vi "dummy encoder edge detection (non-FPGA style).vi"(5 "Tick Count(Ticks)":u32, 6 "rising edge (T)":bool=TRUE, 7 "switch encoders (F)":bool, 8 "ticks":u32[](array[numeric])=[0, 0], 9 "encoder 2":bool, 10 "encoder 1":bool, 11 "history in":bool[](array[boolean])=[FALSE, FALSE, FALSE, FALSE, FALSE, FALSE, FALSE, FALSE, FALSE, FALSE, FALSE, FALSE, FALSE, FALSE, FALSE, FALSE, FALSE, FALSE, FALSE, FALSE, FALSE, FALSE, FALSE, FALSE, FALSE, FALSE, FALSE, FALSE, FALSE, FALSE, FALSE, FALSE, FALSE, FALSE, FALSE, FALSE, FALSE, FALSE, FALSE, FALSE, FALSE, FALSE, FALSE, FALSE, FALSE, FALSE, FALSE, FALSE, FALSE, FALSE, FALSE, FALSE, FALSE, FALSE, FALSE, FALSE, FALSE, FALSE, FALSE, FALSE, FALSE, FALSE, FALSE, FALSE, FALSE, FALSE, FALSE, FALSE, FALSE, FALSE, FALSE, FALSE, FALSE, FALSE, FALSE, FALSE, FALSE, FALSE, FALSE, FALSE, FALSE, FALSE, FALSE, FALSE, FALSE, FALSE, FALSE, FALSE, FALSE, FALSE, FALSE, FALSE, FALSE, FALSE, FALSE, FALSE, FALSE, FALSE, FALSE, FALSE]) -> (0 "ticks out":u32[](array[numeric]), 1 "edge detected":bool, 3 "history out":bool[](array[boolean]))   [LabVIEW 2018]
panel:
  in  "edge rejection length":i16=5
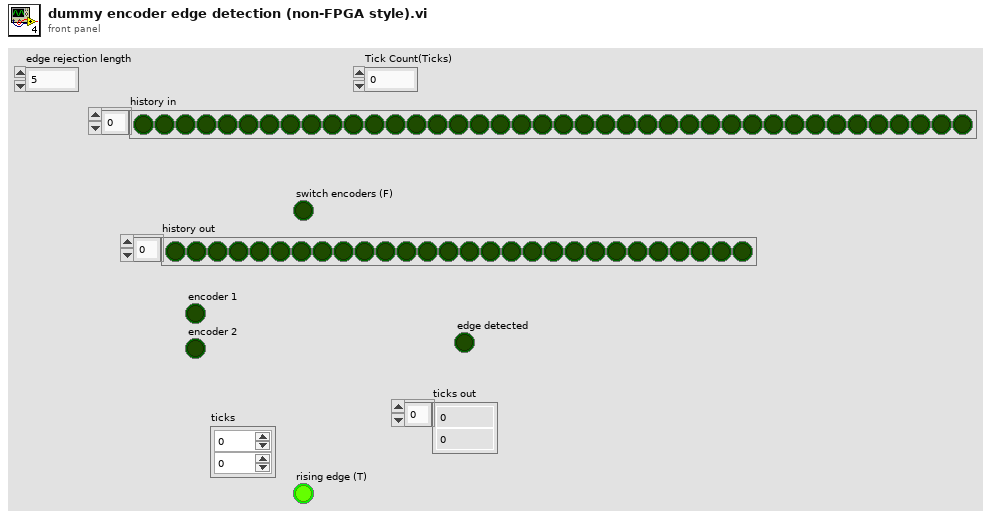
[diagram p1: front panel]
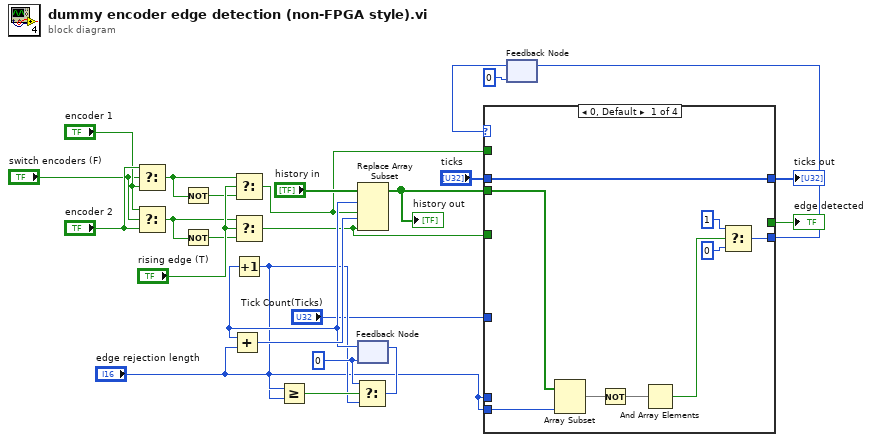
[diagram p0: block diagram]
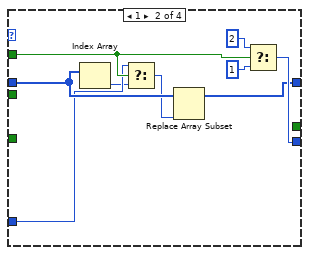
[diagram p2: hidden frame]
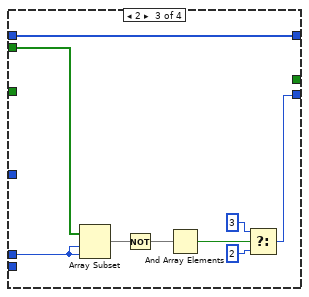
[diagram p3: hidden frame]
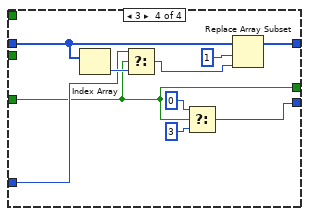
[diagram p4: hidden frame]
diagram:
  w18 = i16 0 ("t")
  n1 = Select(t="encoder 2", s="switch encoders (F)", f="encoder 1") -> (s? t:f=w4:bool)
  n2 = Select(t="encoder 1", s="switch encoders (F)", f="encoder 2") -> (s? t:f=w3:bool)
  n3 = Not(x=w4) -> (.not. x?=w23:bool)
  n4 = Not(x=w3) -> (.not. x?=w22:bool)
  n5 = Select(t=w4, s="rising edge (T)", f=w23) -> (s? t:f=w14:bool)
  n6 = Select(t=w3, s="rising edge (T)", f=w22) -> (s? t:f=w13:bool)
  n7 = feedback #1(w18) -> (w19:i16)
  n8 = Add(x=w19, y="edge rejection length") -> (x+y=w26:i16)
  n9 = Increment(x=w19) -> (x+1=w16:i16)
  n10 = Greater Or Equal?(x=w16, y="edge rejection length") -> (x >= y?=w25:bool)
  n11 = Select(t=w18, s=w25, f=w16) -> (s? t:f=w20:i16)
  n12 = Replace Array Subset(array="history in", new element #1=w14, index #1=w19, new element #2=w13, index #2=w26) -> (w12:bool[])
  "history out" <- w12
  n13 = feedback-in #1(w20) -> ()
  n14 = feedback #2(u8 0 ("f")) -> (w9:u8)
  n15 = case shown="0, Default" w9 {
    tunnel: w12 -> [w33 _ w51 _]
    tunnel: [w30 w43 w47 w62] -> w10
    tunnel: w14 -> [_ w40 _ _]
    tunnel: w13 -> [_ _ _ w54]
    tunnel: "ticks" -> [w28 w42 w46 w59]
    tunnel: [w28 w41 w46 w60] -> w11
    tunnel: "Tick Count(Ticks)" -> [_ w39 _ w56]
    tunnel: [_ _ _ w54] -> w8
    tunnel: "edge rejection length" -> [w27 _ _ _]
    tunnel: "edge rejection length" -> [_ _ w45 _]
    frame 0, Default {
      n16 = Array Subset(array=w33, length=w27) -> (w35:bool[])  [unwired: 1 in]
      n17 = Not(x=w35) -> (.not. x?=w34:bool[])
      n18 = And Array Elements(Boolean array=w34) -> (logical AND=w32:bool)
      n19 = Select(t=u8 1 ("next state"), s=w32, f=u8 0 ("next state")) -> (s? t:f=w30:u8)
    }
    frame 1 {
      n20 = Index Array(array=w42) -> (element=w38:u32)  [unwired: 1 in]
      n21 = Select(t=w39, s=w40, f=w38) -> (s? t:f=w37:u32)
      n22 = Replace Array Subset(array=w42, new element=w37) -> (w41:u32[])  [unwired: 1 in]
      n23 = Select(t=u8 2, s=w40, f=u8 1) -> (s? t:f=w43:u8)
    }
    frame 2 {
      n24 = Array Subset(array=w51, index=w45, length=w45) -> (w53:bool[])
      n25 = Not(x=w53) -> (.not. x?=w52:bool[])
      n26 = And Array Elements(Boolean array=w52) -> (logical AND=w48:bool)
      n27 = Select(t=u8 3, s=w48, f=u8 2) -> (s? t:f=w47:u8)
    }
    frame 3 {
      n28 = Index Array(array=w59) -> (element=w58:u32)  [unwired: 1 in]
      n29 = Select(t=w56, s=w54, f=w58) -> (s? t:f=w57:u32)
      n30 = Select(t=u8 0, s=w54, f=u8 3) -> (s? t:f=w62:u8)
      n31 = Replace Array Subset(array=w59, new element=w57, index=1) -> (w60:u32[])
    }
  }
  "edge detected" <- w8
  "ticks out" <- w11
  n32 = feedback-in #2(w10) -> ()
